vi "logic.vi"() -> ()   [LabVIEW 2013]
panel:
  in  "Boolean":bool
  in  "Chassis has an LED panel":bool
  in  "Number of Slots":i32
  in  "Card Type":T1(array[ring])
  out "Slot #":dbl[](array[numeric])
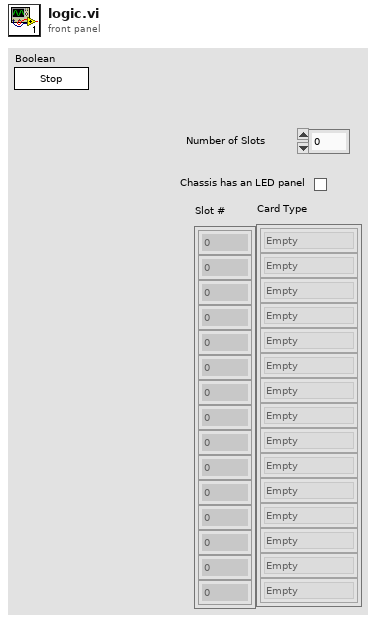
[diagram p1: front panel]
types:
  T1 = enum16{"Empty", "UEGO", "DIO", "Fault Insertion", "Other"}[]
  T2 = enum16{"Empty", "UEGO", "DIO", "Fault Insertion", "Other"}
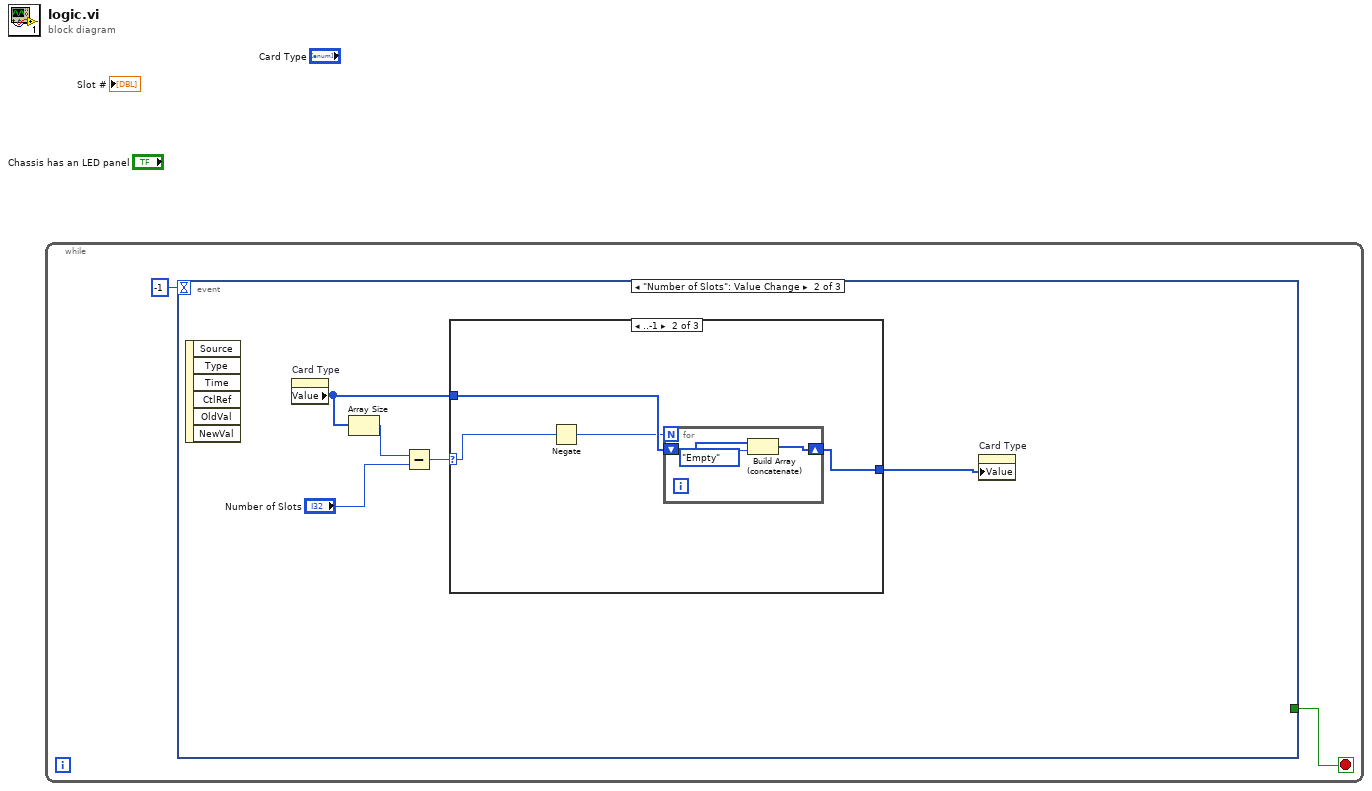
[diagram p0: block diagram]
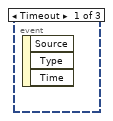
[diagram p2: hidden frame]
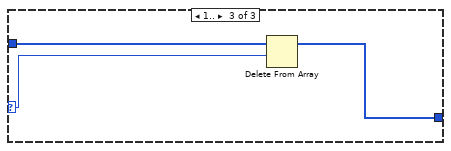
[diagram p4: hidden frame]
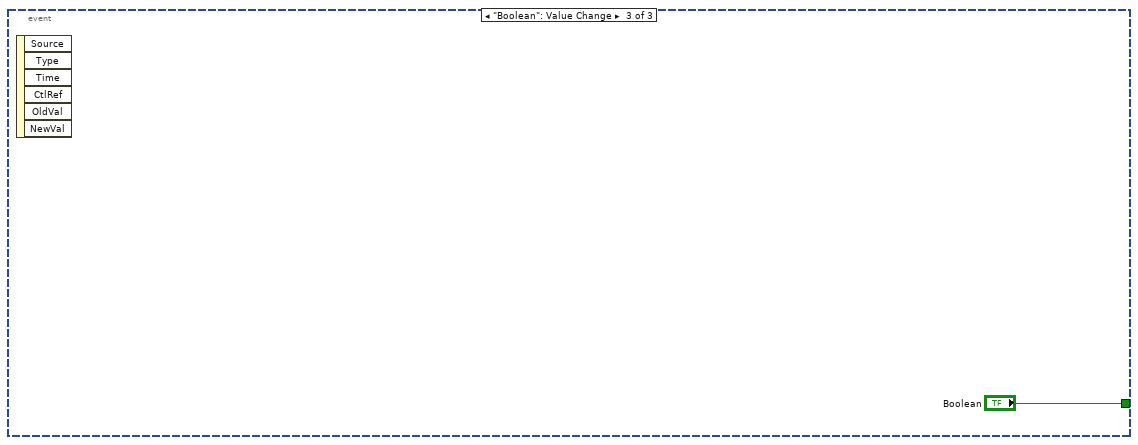
[diagram p5: hidden frame]
diagram:
  n1 = while {
    stop <- w1 stop-if-true
    n2 = event shown="[1] \"Number of Slots\": Value Change" {
      selector: _ -> [_ _ _]
      dyn-events: _ -> [_ _ _]
      timeout: -1 -> [_ _ _]
      tunnel: [_ _ "Boolean"] -> w1
      event Timeout {
        n3 = event-data() -> ()  [unwired: 1 in, 3 out]
      }
      event "Number of Slots": Value Change {
        n4 = event-data() -> ()  [unwired: 1 in, 6 out]
        n5 = property on="Card Type" class="Arr (strict)"() -> ("Value"=w4:T1)  [unwired: 2 in, 2 out]
        n6 = Array Size(array=w4) -> (size(s)=w7:i32)
        n7 = Subtract(x=w7, y="Number of Slots") -> (x-y=w5:i32)
        n8 = case shown="..-1" w5 {
          selector: w5 -> [_ w11 w17]
          tunnel: w4 -> [w8 w12 w18]
          tunnel: [w8 w10 w16] -> w3
          frame 0 {
          }
          frame ..-1 {
            n9 = Negate(x=w11) -> (-x=w9:i32)
            n10 = for {
              N: w9 -> [_]
              shift-right: [w13] -> w10
              shift-left: w12 -> [w15]
              n11 = Build Array (concatenate)(w15, T2."Empty" ("Enum")) -> (w13:T1)
            }
          }
          frame 1.. {
            n12 = Delete From Array(array=w18, length=w17) -> (array with subset deleted=w16:T1)  [unwired: 1 in, 1 out]
          }
        }
        n13 = property on="Card Type" class="Arr (strict)"("Value"=w3) -> ()  [unwired: 2 in, 2 out]
      }
      event "Boolean": Value Change {
        n14 = event-data() -> ()  [unwired: 1 in, 6 out]
      }
    }
  }
